vi "Draw_Cage_Outline_(square)_substep_1.vi"(6 "Color":u32(colorbox)=9868950, 8 "error in (no error)":errorcluster, 9 "Bounding rectangle for cage outline, pix":T2, 10 "Corner scale  factor":dbl, 11 "Refnum in":T1) -> (0 "error out":errorcluster, 3 "Refnum out":T1)   [LabVIEW 2018, in "Cage Diagram.lvlib"]
uses:
  Cage Diagram.lvlib
  <vilib>/vision/Image Controls.llb/IMAQ Image.ctl
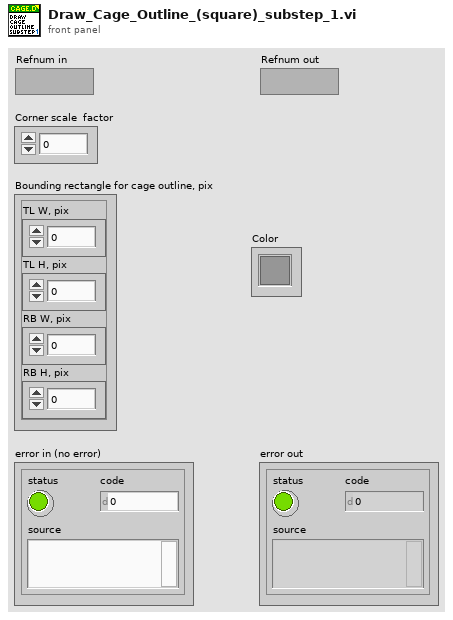
[diagram p1: front panel]
types:
  T1 = typedef "IMAQ Image.ctl" = refnum<image>
  T2 = cluster{"TL W, pix":i32, "TL H, pix":i32, "RB W, pix":i32, "RB H, pix":i32}
  T3 = cluster{"X Left":dbl, "Y Top":dbl, "X Right":dbl, "Y Bottom":dbl}
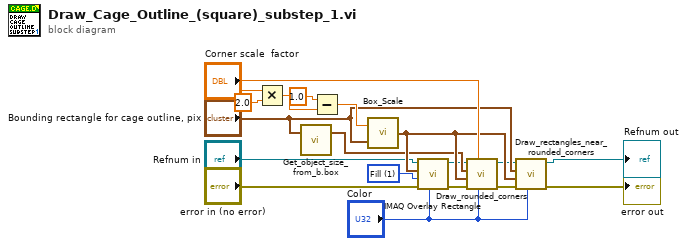
[diagram p0: block diagram]
diagram:
  w6 = u32 1 items=["Frame", "Fill", "Highlight"] ("Drawing Mode (Frame)")
  n1 = Multiply(x="Corner scale  factor", y=2.0) -> (x*y=w17:dbl)
  n2 = call "Get_object_size_from_b.box.vi"("Bounding rectangle for cage outline, pix"="Bounding rectangle for cage outline, pix") -> ("Object Size, pix"=w5:cluster{"W":dbl, "H":dbl})  [unwired: 2 in]
  n3 = Subtract(x=1.0, y=w17) -> (x-y=w14:dbl)
  n4 = call "Box_Scale.vi"("Rectangle in"="Bounding rectangle for cage outline, pix", "Scale factor"=w14) -> ("Rectangle out"=w12:T3)
  n5 = call "IMAQ Overlay Rectangle"("Color"="Color", "error in (no error)"="error in (no error)", "Drawing Mode (Frame)"=w6, "Rectangle"=w12, "Image"="Refnum in") -> ("error out"=w3:errorcluster, "Image Out"=w4:T1)  [unwired: 5 in]
  n6 = call "Draw_rounded_corners.vi"("Color"="Color", "Corner scale  factor"="Corner scale  factor", "error in (no error)"=w3, "Inner box coords"=w12, "Whole cage size, pix"=w5, "Refnum in"=w4) -> ("error out"=w7:errorcluster, "Refnum out"=w10:T1)  [unwired: 4 in]
  n7 = call "Draw_rectangles_near_rounded_corners.vi"("Color"="Color", "error in (no error)"=w7, "Inner box coords"=w12, "Outer box coords"="Bounding rectangle for cage outline, pix", "Refnum in"=w10) -> ("error out"=→"error out":errorcluster, "Refnum out"=→"Refnum out":T1)  [unwired: 5 in]
